vi "parseLaserScan.vi"(4 "error in":errorcluster, 7 "msg in":string) -> (0 "error out":errorcluster, 1 "Bearing Array":dbl[](array[numeric]), 2 "Range Array":sgl[](array[numeric]), 3 "Scan Details":T1)   [LabVIEW 2016]
doc: "Parses a message into a range"
uses:
  <vilib>/Tufts CEEO ROS for LabVIEW Software/ROS/MessageParsing/std_msgs/subs/parse_float32_scalar.vi
panel:
  out "Size Bear.":i32
  out "size Range":i32
  out "msg out":string
  out "Header":T2
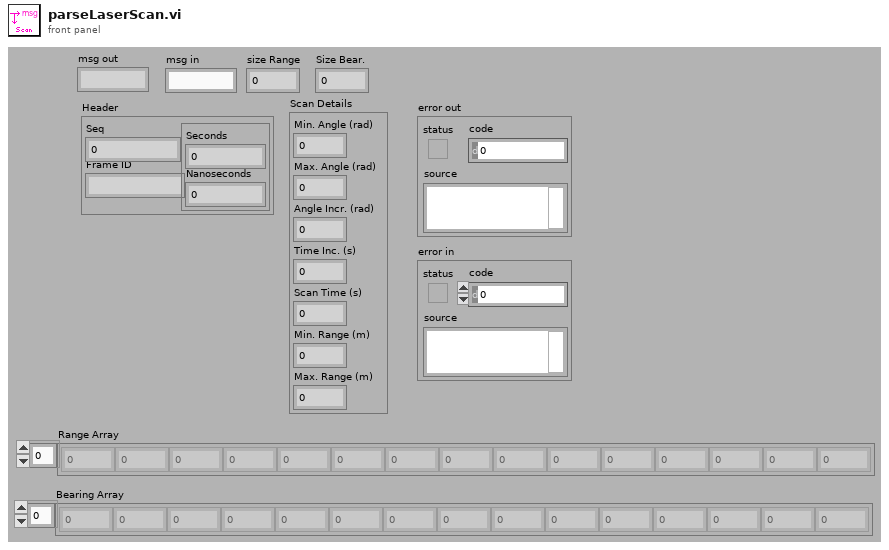
[diagram p1: front panel]
types:
  T1 = cluster{"Min. Angle (rad)":dbl, "Max. Angle (rad)":dbl, "Angle Incr. (rad)":dbl, "Time Inc. (s)":dbl, "Scan Time (s)":dbl, "Min. Range (m)":dbl, "Max. Range (m)":dbl}
  T2 = cluster{"Seq":u32, "Frame ID":string, cluster{"Seconds":i32, "Nanoseconds":i32}}
  T3 = cluster{"Seq":u32, "Frame ID":string, "Timestamp":cluster{"Seconds":i32, "Nanoseconds":i32}}
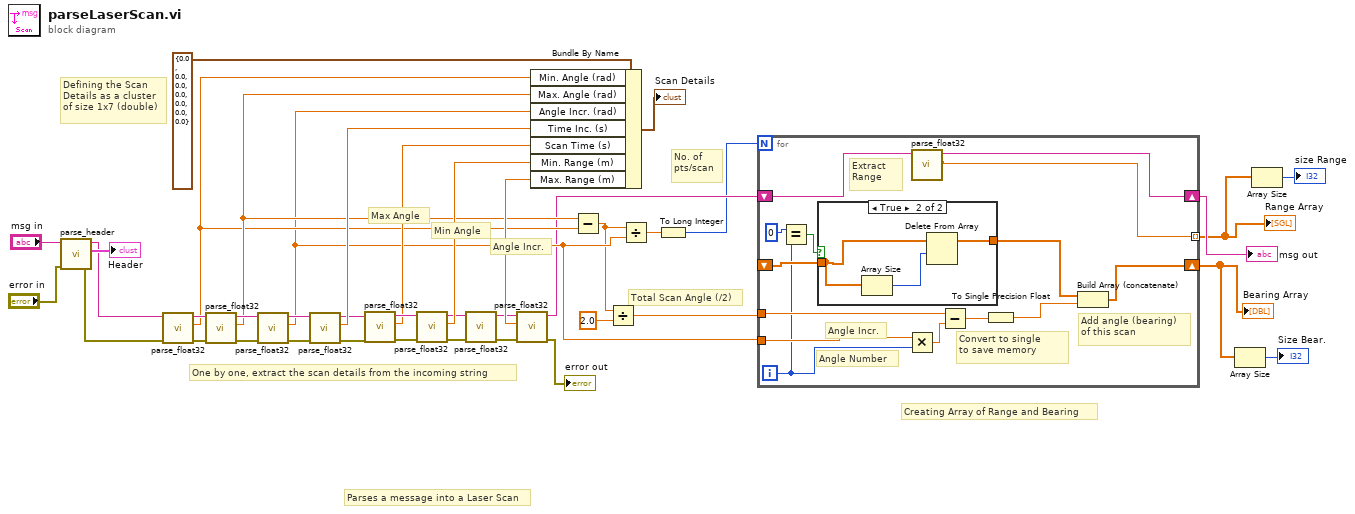
[diagram p0: block diagram]
diagram:
  # "One by one, extract the scan details from the incoming string"
  # "Defining the Scan \nDetails as a cluster \nof size 1x7 (double)"
  # "Total Scan Angle (/2)"
  # "Angle Incr."
  # "Min Angle"
  # "Max Angle"
  # "No. of pts/scan"
  # "Creating Array of Range and Bearing"
  # "Parses a message into a Laser Scan"
  n1 = call <vilib>:"parse_header.vi"("error in"="error in", "msg in"="msg in") -> ("error out"=w30:errorcluster, "Header"=→"Header":T3, "msg out"=w31:string)  [unwired: 3 in]
  n2 = call-poly <vilib>:"parse_float32.vi"("error in"=w30, "msg in"=w31) -> ("error out"=w38:errorcluster, "number"=w17:sgl, "msg out"=w39:string)  [unwired: 3 in]
  n3 = call-poly <vilib>:"parse_float32.vi"("error in"=w38, "msg in"=w39) -> ("error out"=w37:errorcluster, "number"=w18:sgl, "msg out"=w36:string)  [unwired: 3 in]
  n4 = call-poly <vilib>:"parse_float32.vi"("error in"=w37, "msg in"=w36) -> ("error out"=w34:errorcluster, "number"=w16:sgl, "msg out"=w35:string)  [unwired: 3 in]
  n5 = call-poly <vilib>:"parse_float32.vi"("error in"=w34, "msg in"=w35) -> ("error out"=w22:errorcluster, "number"=w28:sgl, "msg out"=w27:string)  [unwired: 3 in]
  n6 = call-poly <vilib>:"parse_float32.vi"("error in"=w22, "msg in"=w27) -> ("error out"=w21:errorcluster, "number"=w25:sgl, "msg out"=w26:string)  [unwired: 3 in]
  n7 = call-poly <vilib>:"parse_float32.vi"("error in"=w21, "msg in"=w26) -> ("error out"=w4:errorcluster, "number"=w24:sgl, "msg out"=w6:string)  [unwired: 3 in]
  n8 = call-poly <vilib>:"parse_float32.vi"("error in"=w4, "msg in"=w6) -> ("error out"=w3:errorcluster, "msg out"=w5:string)  [unwired: 3 in, 1 out]
  n9 = call-poly <vilib>:"parse_float32.vi"("error in"=w3, "msg in"=w5) -> ("error out"=→"error out":errorcluster, "number"=w23:sgl, "msg out"=w15:string)  [unwired: 3 in]
  n10 = Bundle By Name(cluster=T1 {"Min. Angle (rad)"=0.0, "Max. Angle (rad)"=0.0, "Angle Incr. (rad)"=0.0, "Time Inc. (s)"=0.0, "Scan Time (s)"=0.0, "Min. Range (m)"=0.0, "Max. Range (m)"=0.0}, "Min. Angle (rad)"=w17, "Max. Angle (rad)"=w18, "Angle Incr. (rad)"=w16, "Time Inc. (s)"=w28, "Scan Time (s)"=w25, "Min. Range (m)"=w24, "Max. Range (m)"=w23) -> (→"Scan Details":T1)
  n11 = Subtract(x=w18, y=w17) -> (x-y=w8:sgl)
  n12 = Divide(x=w8, y=2.0) -> (x/y=w7:dbl)
  n13 = Divide(x=w8, y=w16) -> (x/y=w2:sgl)
  n14 = To Long Integer(number=w2) -> (32bit integer=w1:i32)
  n15 = for {
    N: w1 -> [_]
    tunnel: w16 -> [w54]
    shift-right: [w53] -> w10
    shift-left: _ -> [w49]
    shift-right: [w51] -> w14
    shift-left: w15 -> [w52]
    tunnel: [w41] -> w13 mode=indexing
    tunnel: w7 -> [w50]
    i -> [w47]
    # "Extract \nRange"
    # "Convert to single\nto save memory"
    # "Angle Number"
    # "Angle Incr."
    # "Add angle (bearing) of this scan"
    n16 = Equal?(x=0, y=w47) -> (x = y?=w48:bool)
    n17 = case shown="True" w48 {
      tunnel: w49 -> [w55 w57]
      tunnel: [w55 w56] -> w45
      frame False {
      }
      frame True {
        n18 = Array Size(array=w57) -> (size(s)=w58:i32)
        n19 = Delete From Array "Delete From Array"(array=w57, length=w58) -> (array with subset deleted=w56:sgl[])  [unwired: 1 in, 1 out]
      }
    }
    n20 = Multiply(x=w54, y=w47) -> (x*y=w44:sgl)
    n21 = call-poly <vilib>:"parse_float32.vi"("msg in"=w52) -> ("number"=w41:sgl, "msg out"=w51:string)  [unwired: 4 in, 1 out]
    n22 = Subtract(x=w50, y=w44) -> (x-y=w43:dbl)
    n23 = To Single Precision Float(number=w43) -> (single precision float=w42:sgl)
    n24 = Build Array (concatenate)(w45, w42) -> (w53:sgl[])
  }
  "Range Array" <- w13
  "Bearing Array" <- w10
  "msg out" <- w14
  n25 = Array Size(array=w10) -> (size(s)=→"Size Bear.":i32)
  n26 = Array Size(array=w13) -> (size(s)=→"size Range":i32)
